vi "CLD3 FGV Timer Exercise.vi"(8 "Error In":errorcluster, 10 "Time Target (s)":dbl=4.0, 11 "Timer Mode":T1) -> (0 "Error Out":errorcluster, 2 "Has Time Elapsed":bool, 3 "Elapsed Time (s.ss)":dbl)   [LabVIEW 2025]
doc: "FGV timer that implements four modes: Start Timer, Read Time, Pause and Resume."
uses:
  CLD3 FGV Mode.ctl
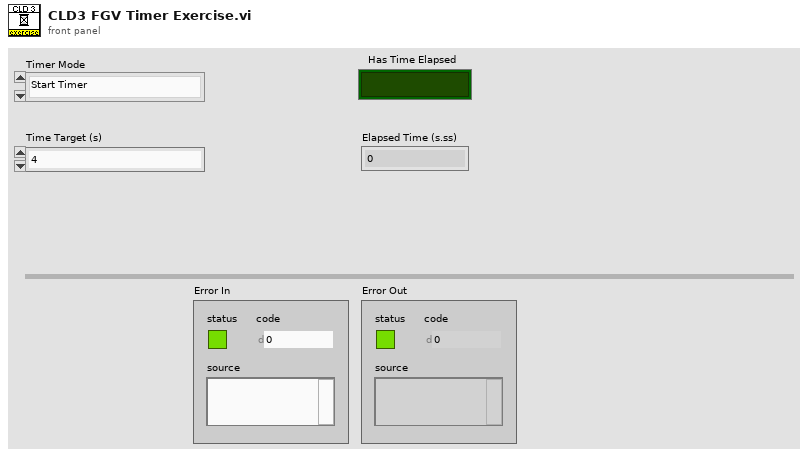
[diagram p1: front panel]
types:
  T1 = typedef "CLD3 FGV Mode.ctl" = enum16{"Start Timer", "Read Time", "Pause", "Resume"}
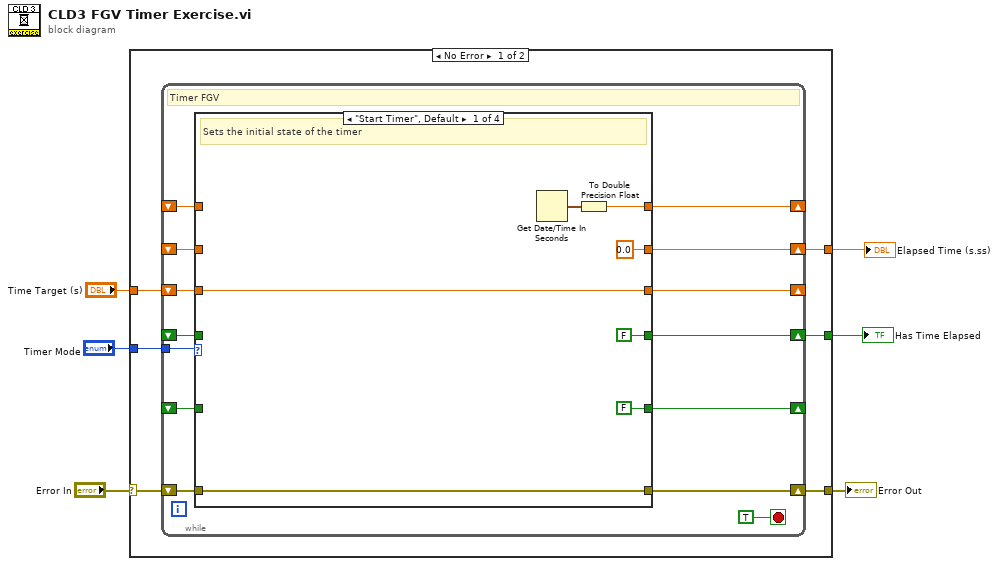
[diagram p0: block diagram]
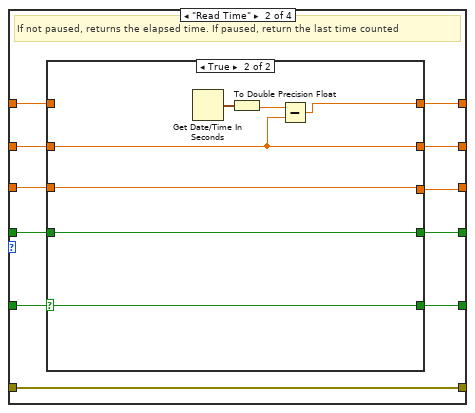
[diagram p2: hidden frame]
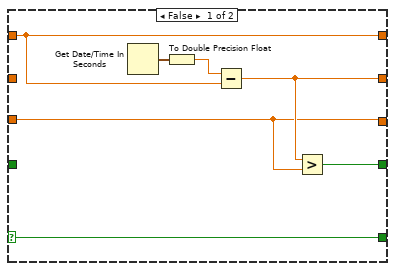
[diagram p3: hidden frame]
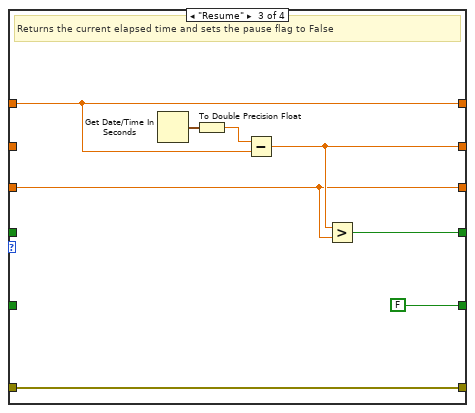
[diagram p4: hidden frame]
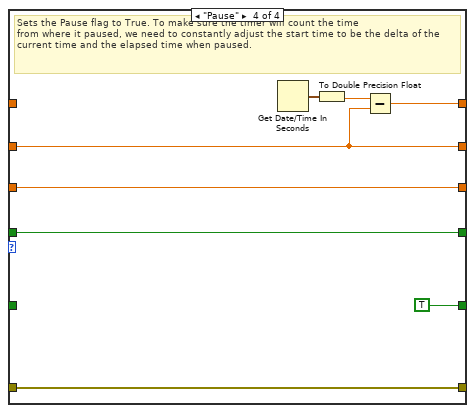
[diagram p5: hidden frame]
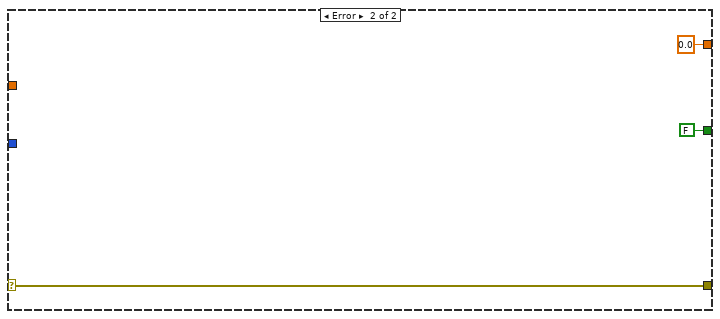
[diagram p6: hidden frame]
diagram:
  n1 = case shown="No Error" "Error In" {
    selector: "Error In" -> [w12 w77]
    tunnel: [w11 w77] -> w5
    tunnel: "Timer Mode" -> [w10 _]
    tunnel: "Time Target (s)" -> [w9 _]
    tunnel: [w8 0.0 ("Elapsed Time (s.ss)")] -> w2
    tunnel: [w7 FALSE] -> w1
    frame No Error {
      n2 = while {
        shift-right: [w25] -> w11
        shift-left: w12 -> [w26]
        tunnel: w10 -> [w23]
        shift-right: [w21] -> _
        shift-left: w9 -> [w22]
        shift-right: [w19] -> _
        shift-left: _ -> [w18]
        shift-right: [w20] -> w8
        shift-left: _ -> [w16]
        shift-right: [w17] -> w7
        shift-left: _ -> [w15]
        shift-right: [w14] -> _
        shift-left: _ -> [w13]
        stop <- TRUE stop-if-true
        # "Timer FGV"
        n3 = case shown="\"Start Timer\", Default" w23 {
          tunnel: w26 -> [w29 w44 w66 w74]
          tunnel: [w29 w44 w66 w74] -> w25
          tunnel: w22 -> [w33 w41 w62 w73]
          tunnel: [w33 w36 w62 w73] -> w21
          tunnel: [0.0 ("Elapsed Time (s.ss)") w42 w65 w69] -> w20
          tunnel: [w30 w37 w61 w68] -> w19
          tunnel: w18 -> [_ w43 w61 _]
          tunnel: [FALSE w40 w64 w72] -> w17
          tunnel: w16 -> [_ w35 _ w69]
          tunnel: w15 -> [_ w34 _ w72]
          tunnel: [FALSE w38 FALSE TRUE] -> w14
          tunnel: w13 -> [_ w39 _ _]
          frame "Start Timer", Default {
            # "Sets the initial state of the timer"
            n4 = Get Date/Time In Seconds() -> (seconds since 1Jan1904=w31:timestamp)
            n5 = To Double Precision Float(number=w31) -> (double precision float=w30:dbl)
          }
          frame "Read Time" {
            # "If not paused, returns the elapsed time. If paused, return the last time counted"
            n6 = case shown="True" w39 {
              selector: w39 -> [w47 w56]
              tunnel: w43 -> [w46 _]
              tunnel: [w49 w53] -> w42
              tunnel: w41 -> [w45 w58]
              tunnel: [w48 w57] -> w40
              tunnel: [w47 w56] -> w38
              tunnel: [w46 w52] -> w37
              tunnel: [w45 w58] -> w36
              tunnel: w35 -> [_ w53]
              tunnel: w34 -> [_ w57]
              frame False {
                n7 = Get Date/Time In Seconds() -> (seconds since 1Jan1904=w51:timestamp)
                n8 = To Double Precision Float(number=w51) -> (double precision float=w50:dbl)
                n9 = Subtract(x=w50, y=w46) -> (x-y=w49:dbl)
                n10 = Greater?(x=w49, y=w45) -> (0:w48:bool)
              }
              frame True {
                n11 = Get Date/Time In Seconds() -> (seconds since 1Jan1904=w55:timestamp)
                n12 = To Double Precision Float(number=w55) -> (double precision float=w54:dbl)
                n13 = Subtract(x=w54, y=w53) -> (x-y=w52:dbl)
              }
            }
          }
          frame "Resume" {
            # "Returns the current elapsed time and sets the pause flag to False"
            n14 = Get Date/Time In Seconds() -> (seconds since 1Jan1904=w60:timestamp)
            n15 = To Double Precision Float(number=w60) -> (double precision float=w59:dbl)
            n16 = Subtract(x=w59, y=w61) -> (x-y=w65:dbl)
            n17 = Greater?(x=w65, y=w62) -> (0:w64:bool)
          }
          frame "Pause" {
            # "Sets the Pause flag to True. To make sure the timer will count the time\nfrom where it paused, we need to constantly adjust the start time to be the delta of the current time and the elapsed time when paused."
            n18 = Get Date/Time In Seconds() -> (seconds since 1Jan1904=w71:timestamp)
            n19 = To Double Precision Float(number=w71) -> (double precision float=w70:dbl)
            n20 = Subtract(x=w70, y=w69) -> (x-y=w68:dbl)
          }
        }
      }
    }
    frame Error {
    }
  }
  "Error Out" <- w5
  "Elapsed Time (s.ss)" <- w2
  "Has Time Elapsed" <- w1
